vi "Start Vecto.vi"(8 "error in (no error)":errorcluster, 11 "VolatusCore in":refnum<class "VolatusCore.lvclass">) -> (0 "error out":errorcluster, 3 "VolatusCore out":refnum<class "VolatusCore.lvclass">)   [LabVIEW 2020, in "Volatus.lvlib" / "VolatusCore.lvclass"]
uses:
  VolatusCore.lvclass
  VolatusCore.lvclass/VolatusCore.ctl
  lv-vecto/Vecto/Vecto/Vecto.lvclass
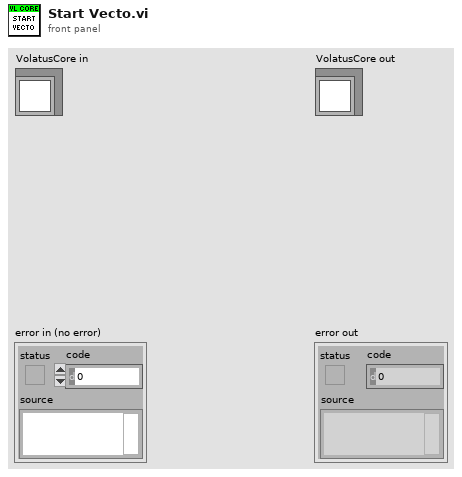
[diagram p1: front panel]
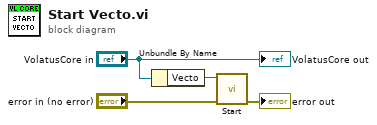
[diagram p0: block diagram]
diagram:
  n1 = Unbundle By Name("VolatusCore in") -> ("Vecto"=w4:refnum<class "Vecto.lvclass">)
  n2 = call "Start.vi"("error in (no error)"="error in (no error)", "Vecto in"=w4) -> ("error out"=→"error out":errorcluster)  [unwired: 8 in, 1 out]
  "VolatusCore out" <- "VolatusCore in"
